vi "TableToXYGraph.vi"(1 "Input Table":string[][](array[string])) -> (0 "XY Graph":cluster{"Y":dbl[], "Y":dbl[]}[](graph) caption="Graphe XY")   [LabVIEW 2010]
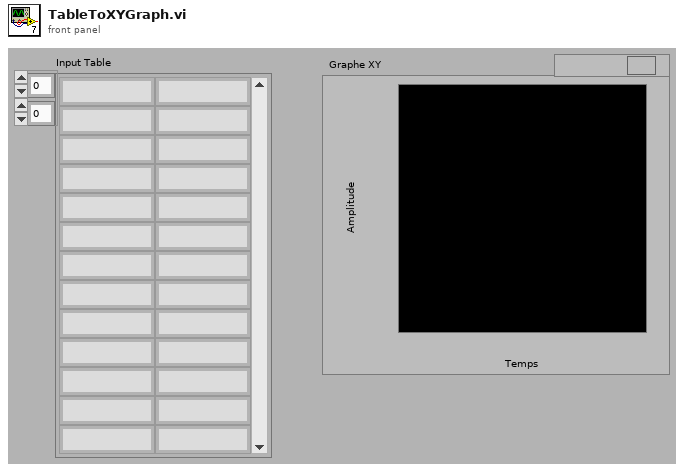
[diagram p1: front panel]
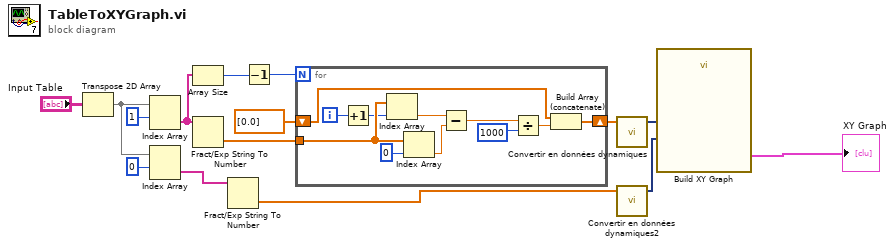
[diagram p0: block diagram]
diagram:
  n1 = Transpose 2D Array(2D array="Input Table") -> (transposed array=w3:string[][])
  n2 = Index Array(array=w3, index (row)=1 ("indice (ligne)")) -> (element=w10:string[])  [unwired: 1 in]
  n3 = Index Array(array=w3, index (row)=0 ("indice (ligne)")) -> (element=w1:string[])  [unwired: 1 in]
  n4 = Array Size(array=w10) -> (size(s)=w11:i32)
  n5 = Fract/Exp String To Number(string=w10) -> (number=w8:dbl[])  [unwired: 3 in, 1 out]
  n6 = Fract/Exp String To Number(string=w1) -> (number=w13:dbl[])  [unwired: 3 in, 1 out]
  n7 = Decrement(x=w11) -> (x-1=w12:i32)
  n8 = for {
    N: w12 -> [_]
    tunnel: w8 -> [w26]
    shift-right: [w16] -> w14
    shift-left: dbl[] [0.0] -> [w17]
    i -> [w25]
    n9 = Increment(x=w25) -> (x+1=w24:i32)
    n10 = Index Array(array=w26, index=w24) -> (element=w22:dbl)
    n11 = Index Array(array=w26, index=0 ("indice")) -> (element=w21:dbl)
    n12 = Subtract(x=w22, y=w21) -> (x-y=w20:dbl)
    n13 = Divide(x=w20, y=1000) -> (x/y=w18:dbl)
    n14 = Build Array (concatenate)(w17, w18) -> (w16:dbl[])
  }
  n15 = call "Convertir en données dynamiques"("Array"=w14) -> ("Dynamic Data Type"=w15:dynamicdata)  [unwired: 3 in]
  n16 = call "Convertir en données dynamiques2"("Array"=w13) -> ("Dynamic Data Type"=w7:dynamicdata)  [unwired: 3 in]
  n17 = call "Build XY Graph"("Y Input"=w7, "X Input"=w15) -> ("XY Graph"=→"XY Graph":cluster{"Y":dbl[], "Y":dbl[]}[])  [unwired: 3 in, 6 out]
